vi "Forward Kinematics.vi"   [LabVIEW 2017, in "NI_Kinematics.lvlib"]
doc: "Returns a homogenous transform or transforms that represents the position of a robotic arm end effector given the joint angles of the arm. Wire data to the <B>joint positions</B> input to determine the polymorphic instance to use or manually select the instance.\n\n<B>.m file:</B> fkine"
uses:
  <vilib>/robotics/Kinematics/NI_Kinematics.lvlib
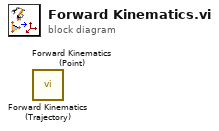
[diagram p0: block diagram]
diagram:
  n1 = call <vilib>:"Forward Kinematics (Trajectory).vi"() -> ()  [unwired: 9 in, 3 out]
  n2 = call <vilib>:"Forward Kinematics (Point).vi"() -> ()  [unwired: 9 in, 3 out]
